vi "Edit Devices Menu View.vi"(8 "error in":errorcluster) -> (0 "error out":errorcluster)   [LabVIEW 2024, in "User Interface.lvlib"]
uses:
  User Interface.lvlib
  Support/General Type Defs/Global Data.vi
  Support/General Type Defs/General Type Definitions.lvlib
panel:
  out "Visualization":string
  in  "IP Address pt2":bool caption="IP Address"
  in  "Alias pt2":bool caption="Alias"
  in  "Hostname pt2":bool caption="Hostname"
  in  "IP Address pt1":bool caption="IP Address"
  in  "Alias pt1":bool caption="Alias"
  in  "Hostname pt1":bool caption="Hostname"
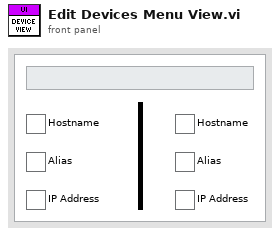
[diagram p1: front panel]
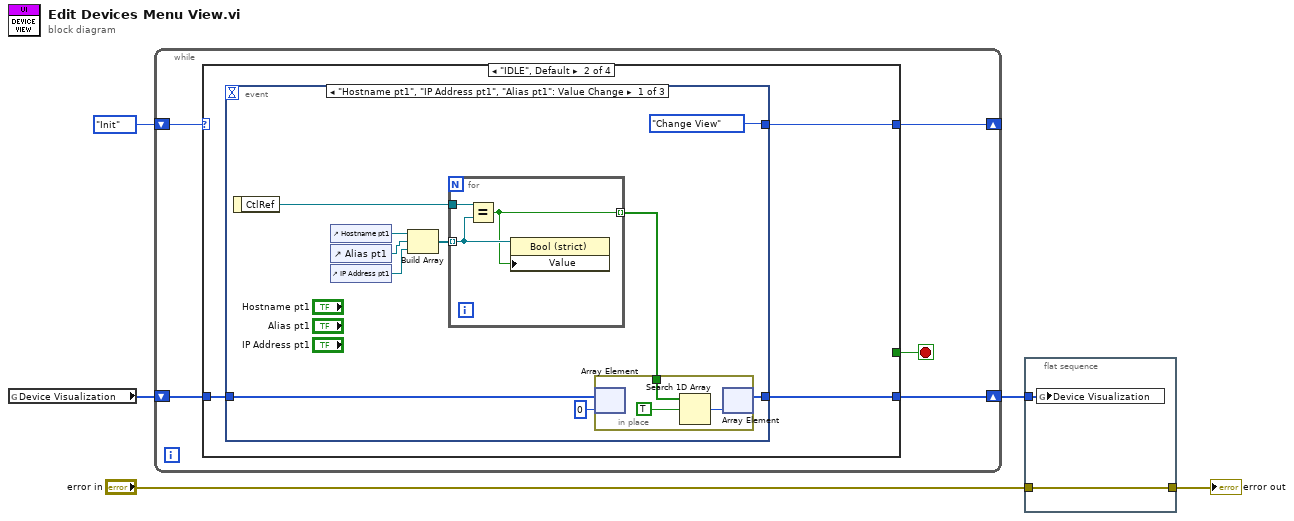
[diagram p0: block diagram]
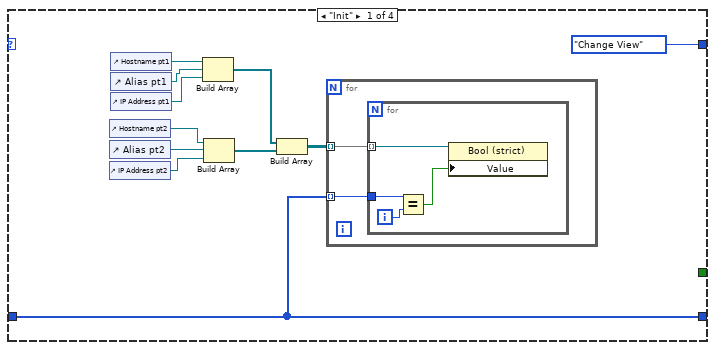
[diagram p2: hidden frame]
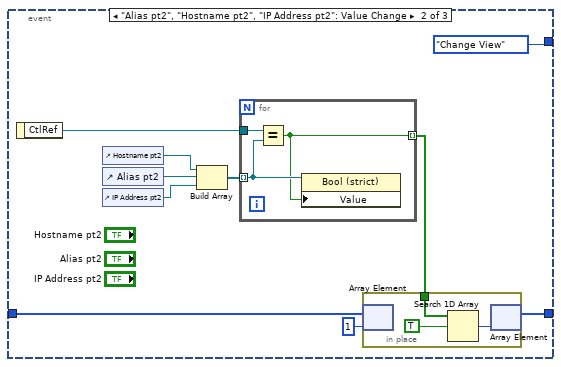
[diagram p3: hidden frame]
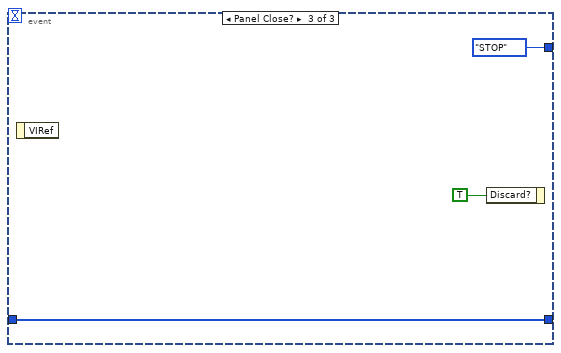
[diagram p4: hidden frame]
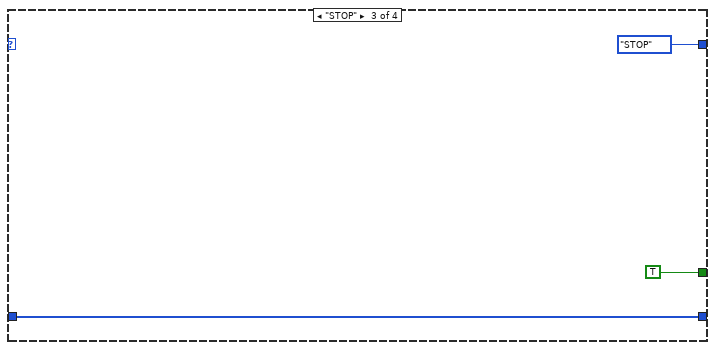
[diagram p5: hidden frame]
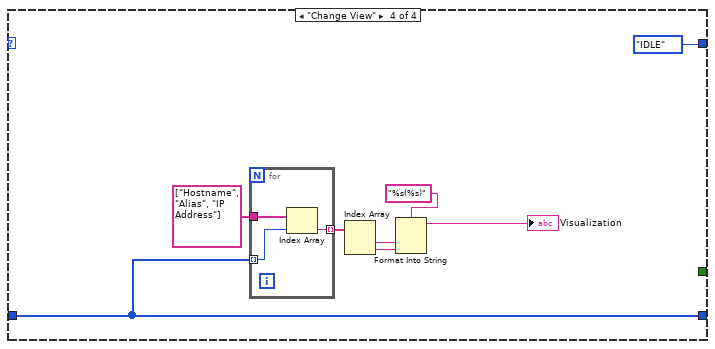
[diagram p6: hidden frame]
diagram:
  n1 = global read "Global Data.vi" "Device Visualization"() -> (w5:i32[])
  n2 = while {
    shift-right: [w9] -> w3
    shift-left: w5 -> [w10]
    shift-right: [w7] -> _
    shift-left: enum16{"Init", "IDLE", "Change View", "STOP"}."Init" -> [w8]
    stop <- w6 stop-if-true
    n3 = case shown="\"IDLE\", Default" w8 {
      tunnel: w10 -> [w11 w30 w68 w70]
      tunnel: [w11 w29 w68 w70] -> w9
      tunnel: [enum16{"Init", "IDLE", "Change View", "STOP"}."Change View" w28 enum16{"Init", "IDLE", "Change View", "STOP"}."STOP" enum16{"Init", "IDLE", "Change View", "STOP"}."IDLE"] -> w7
      tunnel: [_ _ TRUE _] -> w6
      frame "Init" {
        n4 = control-ref of="Hostname pt2"() -> (w17:refnum<vi>)
        n5 = control-ref of="Alias pt2"() -> (w16:refnum<vi>)
        n6 = control-ref of="IP Address pt2"() -> (w18:refnum<vi>)
        n7 = control-ref of="Hostname pt1"() -> (w14:refnum<vi>)
        n8 = control-ref of="Alias pt1"() -> (w13:refnum<vi>)
        n9 = control-ref of="IP Address pt1"() -> (w15:refnum<vi>)
        n10 = Build Array(w14, w13, w15) -> (w19:refnum<vi>[])
        n11 = Build Array(w17, w16, w18) -> (w20:refnum<vi>[])
        n12 = Build Array(w19, w20) -> (w12:refnum<vi>[][])
        n13 = for {
          tunnel: w12 -> [w23] mode=indexing
          tunnel: w11 -> [w22] mode=indexing
          n14 = for {
            tunnel: w23 -> [w25] mode=indexing
            tunnel: w22 -> [w26]
            i -> [w27]
            n15 = Equal?(x=w26, y=w27) -> (x = y?=w24:bool)
            n16 = property class="Bool (strict)"(reference=w25, "Value"=w24) -> ()  [unwired: 1 in, 2 out]
          }
        }
      }
      frame "IDLE", Default {
        n17 = event shown="[0] \"Hostname pt1\", \"IP Address pt1\", \"Alias pt1\": Value Change" {
          selector: _ -> [_ _ _]
          dyn-events: _ -> [_ _ _]
          timeout: _ -> [_ _ _]
          tunnel: w30 -> [w33 w54 w63]
          tunnel: [w34 w52 w63] -> w29
          tunnel: [enum16{"Init", "IDLE", "Change View", "STOP"}."Change View" enum16{"Init", "IDLE", "Change View", "STOP"}."Change View" enum16{"Init", "IDLE", "Change View", "STOP"}."STOP"] -> w28
          event "Hostname pt1", "IP Address pt1", "Alias pt1": Value Change {
            n18 = event-data() -> ("CtlRef"=w38:refnum<vi>)  [unwired: 1 in]
            n19 = control-ref of="Hostname pt1"() -> (w37:refnum<vi>)
            n20 = control-ref of="Alias pt1"() -> (w36:refnum<vi>)
            n21 = control-ref of="IP Address pt1"() -> (w40:refnum<vi>)
            n22 = Build Array(w37, w36, w40) -> (w39:refnum<vi>[])
            n23 = for {
              tunnel: w39 -> [w45] mode=indexing
              tunnel: w38 -> [w46]
              tunnel: [w44] -> w32 mode=indexing
              n24 = Equal?(x=w46, y=w45) -> (x = y?=w44:bool)
              n25 = property class="Bool (strict)"(reference=w45, "Value"=w44) -> ()  [unwired: 1 in, 2 out]
            }
            n26 = in-place {
              in-place-border: w32 -> [w41]
              n27 = in-place-array #1(w33, 0) -> ()  [unwired: 1 out]
              n28 = Search 1D Array(1D array=w41, element=TRUE) -> (index of element=w42:i32)  [unwired: 1 in]
              n29 = in-place-array #1(w42) -> (w34:i32[])  [unwired: 1 out]
            }
          }
          event "Alias pt2", "Hostname pt2", "IP Address pt2": Value Change {
            n30 = event-data() -> ("CtlRef"=w51:refnum<vi>)  [unwired: 1 in]
            n31 = control-ref of="Hostname pt2"() -> (w49:refnum<vi>)
            n32 = control-ref of="Alias pt2"() -> (w48:refnum<vi>)
            n33 = control-ref of="IP Address pt2"() -> (w55:refnum<vi>)
            n34 = Build Array(w49, w48, w55) -> (w56:refnum<vi>[])
            n35 = for {
              tunnel: w56 -> [w58] mode=indexing
              tunnel: w51 -> [w59]
              tunnel: [w57] -> w50 mode=indexing
              n36 = Equal?(x=w59, y=w58) -> (x = y?=w57:bool)
              n37 = property class="Bool (strict)"(reference=w58, "Value"=w57) -> ()  [unwired: 1 in, 2 out]
            }
            n38 = in-place {
              in-place-border: w50 -> [w60]
              n39 = in-place-array #2(w54, 1) -> ()  [unwired: 1 out]
              n40 = Search 1D Array(1D array=w60, element=TRUE) -> (index of element=w61:i32)  [unwired: 1 in]
              n41 = in-place-array #2(w61) -> (w52:i32[])  [unwired: 1 out]
            }
          }
          event Panel Close? {
            n42 = event-data() -> ()  [unwired: 1 in, 1 out]
            n43 = event-data("Discard?"=TRUE) -> ()  [unwired: 1 in, 1 out]
          }
        }
      }
      frame "STOP" {
      }
      frame "Change View" {
        n44 = for {
          tunnel: w70 -> [w78] mode=indexing
          tunnel: string[] ["Hostname", "Alias", "IP Address"] -> [w79]
          tunnel: [w77] -> w73 mode=indexing
          n45 = Index Array(array=w79, index=w78) -> (element=w77:string)
        }
        n46 = Index Array(array=w73) -> (element #1=w74:string, element #2=w75:string)  [unwired: 2 in]
        n47 = Format Into String(format string="%s(%s)", w74, w75) -> (resulting string=→"Visualization":string)  [unwired: 2 in, 1 out]
      }
    }
  }
  n48 = flat-sequence {
    tunnel: w3 -> [w81]
    tunnel: "error in" -> [w80]
    tunnel: [w80] -> w1
    frame #0 {
      n49 = global write "Global Data.vi" "Device Visualization"(w81) -> ()
    }
  }
  "error out" <- w1
